vi "File reader.vi"() -> ()   [LabVIEW 2018]
panel:
  out "output 3":dbl
  out "output 2":dbl
  out "Numero out":dbl
  out "offset past match":i32
  out "after substring":string
  out "match substring":string
  out "before substring":string
  out "text":string
  out "path":path
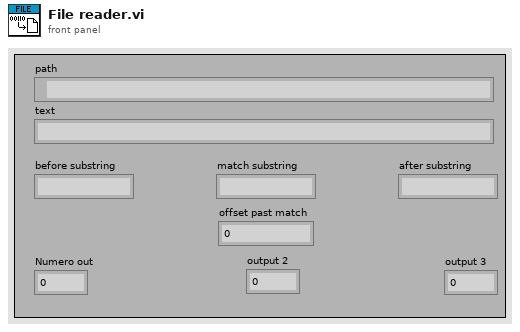
[diagram p1: front panel]
types:
  T1 = enum16{"open", "replace", "create", "open or create", "replace or create", "replace or create with confirmation"}
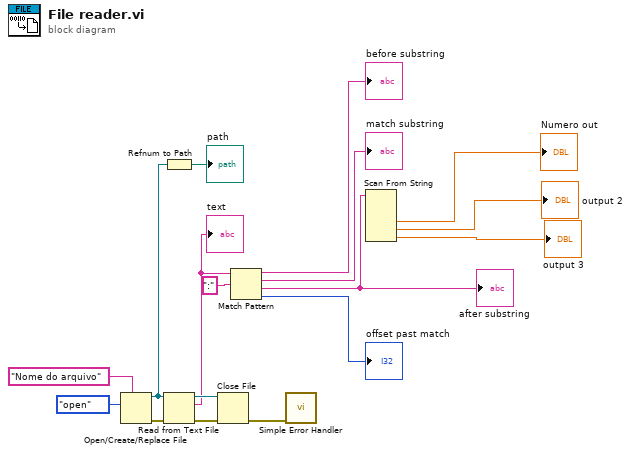
[diagram p0: block diagram]
diagram:
  n1 = Open/Create/Replace File(prompt="Nome do arquivo", operation (0:open)=T1."open") -> (refnum out=w11:refnum<file>, error out=w16:errorcluster)  [unwired: 4 in, 1 out]
  n2 = Refnum to Path(1:w11) -> (0:→"path":path)
  n3 = Read from Text File(file (use dialog)=w11, error in=w16) -> (refnum out=w17:refnum<file>, text=w3:string, error out=w15:errorcluster)  [unwired: 2 in, 1 out]
  "text" <- w3
  n4 = Close File(refnum=w17, error in=w15) -> (error out=w14:errorcluster)  [unwired: 1 out]
  n5 = Match Pattern(string=w3, regular expression=":") -> (before substring=→"before substring":string, match substring=→"match substring":string, after substring=w5:string, offset past match=→"offset past match":i32)  [unwired: 1 in]
  "after substring" <- w5
  n6 = call <vilib>:"Simple Error Handler.vi"("error in (no error)"=w14) -> ()  [unwired: 4 in, 5 out]
  n7 = Scan From String(input string=w5) -> (output 1=→"Numero out":dbl, output 2=→"output 2":dbl, output 3=→"output 3":dbl)  [unwired: 6 in, 3 out]
